vi "User_Event_FGV.vi"(6 "Method":T2(ring), 8 "error in":errorcluster, 11 "User Event":T1) -> (0 "error out":errorcluster, 3 "User Event Out":refnum<user-event>)   [LabVIEW 2020]
uses:
  Def/User_Event.ctl
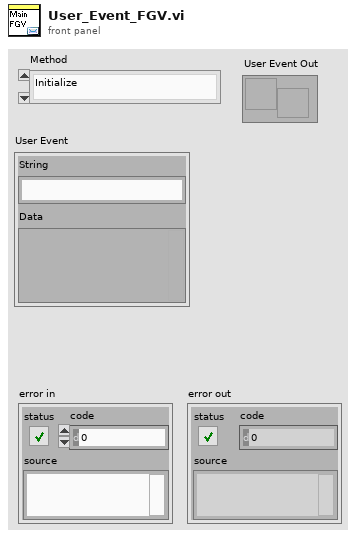
[diagram p1: front panel]
types:
  T1 = typedef "User_Event.ctl" = cluster{"String":string, "Data":variant}
  T2 = enum16{"Initialize", "Get", "Read", "Write", "Release"}
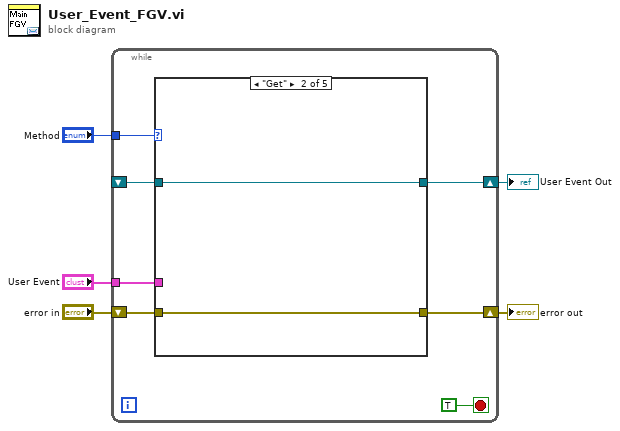
[diagram p0: block diagram]
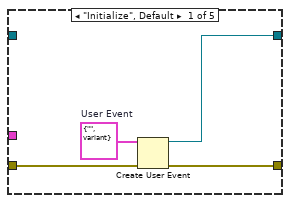
[diagram p2: hidden frame]
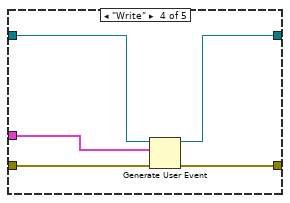
[diagram p4: hidden frame]
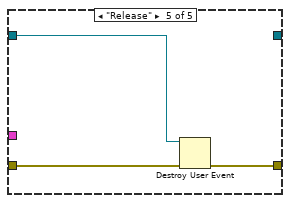
[diagram p5: hidden frame]
diagram:
  n1 = while {
    shift-right: [w10] -> w4
    shift-left: "error in" -> [w11]
    shift-right: [w9] -> w1
    shift-left: _ -> [w8]
    tunnel: "User Event" -> [w7]
    tunnel: "Method" -> [w6]
    stop <- TRUE stop-if-true
    n2 = case shown="\"Get\"" w6 {
      tunnel: w11 -> [w15 w17 w20 w24 w28]
      tunnel: [w14 w17 w20 w23 w27] -> w10
      tunnel: [w13 w18 w19 w22 _] -> w9
      tunnel: w8 -> [_ w18 w19 w25 w26]
      tunnel: w7 -> [_ _ _ w21 _]
      frame "Initialize", Default {
        w16 = T1 {"String"="", "Data"=variant}  # User Event
        n3 = Create User Event(user event datatype=w16, error in=w15) -> (user event=w13:refnum<user-event>, error out=w14:errorcluster)
      }
      frame "Get" {
      }
      frame "Read" {
      }
      frame "Write" {
        n4 = Generate User Event(user event=w25, event data cluster=w21, error in=w24) -> (user event out=w22:refnum<user-event>, error out=w23:errorcluster)  [unwired: 1 in]
      }
      frame "Release" {
        n5 = Destroy User Event(user event=w26, error in=w28) -> (error out=w27:errorcluster)
      }
    }
  }
  "error out" <- w4
  "User Event Out" <- w1
